vi "visionAngleDistance.vi"(11 "Limelight name":string) -> (1 "tvert":dbl, 2 "thor":dbl, 3 "ty":dbl, 4 "ta":dbl)   [LabVIEW 2019]
uses:
  TypeDefs/VisionPipeline.ctl
  ArgosLib/Signal Processing/TypeDefs/EdgeDetector_Type.ctl
  <vilib>/Rock Robotics/Network Tables/NT Write Number.vi
  <vilib>/Rock Robotics/Network Tables/NT Read Number.vi
  ArgosLib/ArgosLib.lvlib
panel:
  out "millisecond timer value":u32
  in  "pipeline control":T1=enum."NoZoom"
  in  "LED control":dbl=3.0 min=0.0 max=3.0
  out "Distance (Area-T_vertical)[In.]":dbl
  out "tx":dbl
  out "Distance (Angle.)[In.]":dbl
  in  "Target Height[in.]":dbl=100.0
  in  "Camera Height[in.]":dbl=30.0
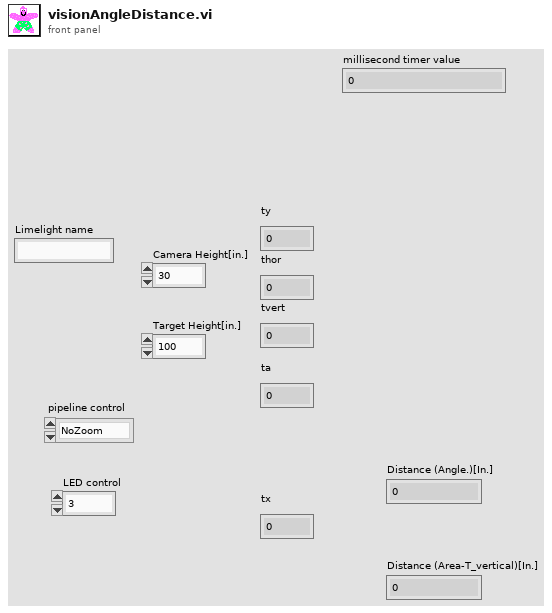
[diagram p1: front panel]
types:
  T1 = typedef "VisionPipeline.ctl" = enum16{"LEDOff", "NoZoom", "Zoom2x", "Zoom3x"}
  T2 = typedef "ArgosLib.lvlib/EdgeDetector_Type.ctl" = enum16{"RisingEdge", "FallingEdge", "Both"}
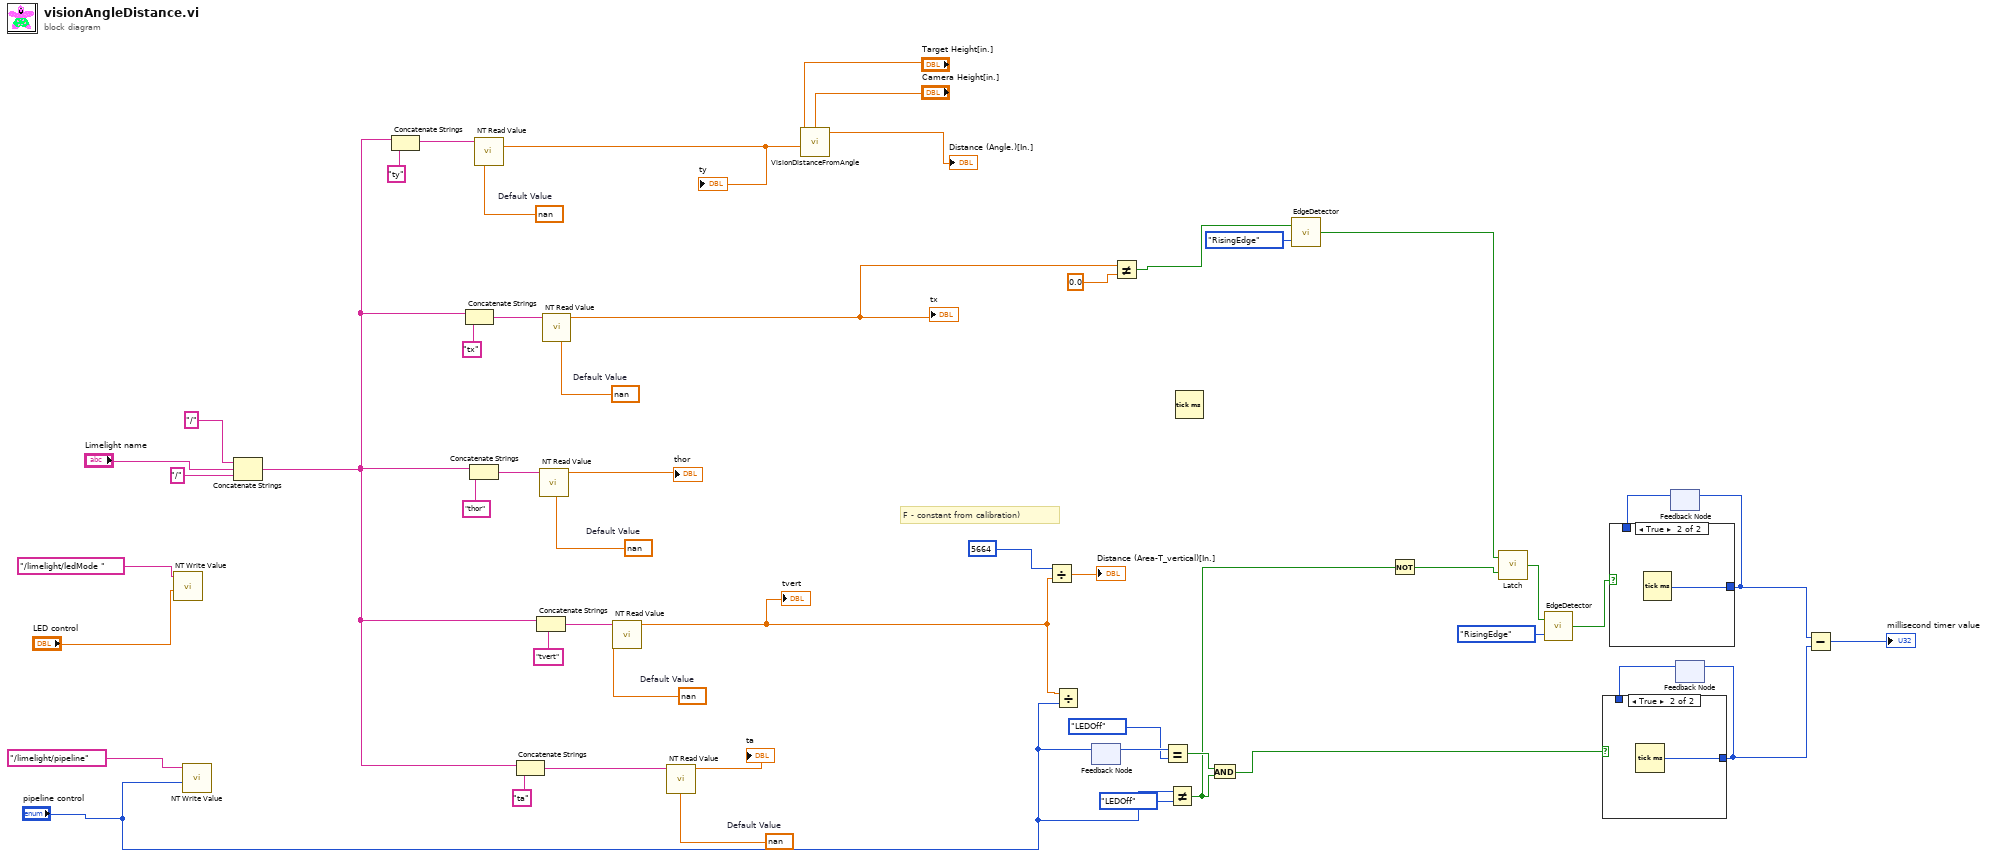
[diagram p0: block diagram]
diagram:
  w34 = nan  # Default Value
  w52 = nan  # Default Value
  w50 = nan  # Default Value
  w49 = nan  # Default Value
  w48 = nan  # Default Value
  # "F - constant from calibration)"
  n1 = call-poly <vilib>:"NT Write Value.vi"("Numeric"="LED control", "Name"="/limelight/ledMode ") -> ()  [unwired: 9 in, 1 out]
  n2 = call-poly <vilib>:"NT Write Value.vi"("Numeric"="pipeline control", "Name"="/limelight/pipeline") -> ()  [unwired: 9 in, 1 out]
  n3 = Concatenate Strings("/" ("string"), "Limelight name", "/" ("string")) -> (w30:string)
  n4 = Concatenate Strings(w30, "ty" ("Name")) -> (w32:string)
  n5 = Concatenate Strings(w30, "tx" ("Name")) -> (w36:string)
  n6 = Concatenate Strings(w30, "thor" ("Name")) -> (w43:string)
  n7 = call-poly <vilib>:"NT Read Value.vi"("Default Value"=w48, "Name"=w32) -> ("Numeric"=w29:dbl)  [unwired: 8 in, 1 out]
  "ty" <- w29
  n8 = Concatenate Strings(w30, "ta" ("Name")) -> (w39:string)
  n9 = Concatenate Strings(w30, "tvert" ("Name")) -> (w41:string)
  n10 = call-poly <vilib>:"NT Read Value.vi"("Default Value"=w49, "Name"=w43) -> ("Numeric"=→"thor":dbl)  [unwired: 8 in, 1 out]
  n11 = call-poly <vilib>:"NT Read Value.vi"("Default Value"=w34, "Name"=w36) -> ("Numeric"=w1:dbl)  [unwired: 8 in, 1 out]
  "tx" <- w1
  n12 = call-poly <vilib>:"NT Read Value.vi"("Default Value"=w50, "Name"=w41) -> ("Numeric"=w24:dbl)  [unwired: 8 in, 1 out]
  "tvert" <- w24
  n13 = call-poly <vilib>:"NT Read Value.vi"("Default Value"=w52, "Name"=w39) -> ("Numeric"=→"ta":dbl)  [unwired: 8 in, 1 out]
  n14 = call "VisionDistanceFromAngle.vi"("Ty"=w29, "Camera Height[in.]"="Camera Height[in.]", "Target Height[in.]"="Target Height[in.]") -> ("Dist. From Target[in.]"=→"Distance (Angle.)[In.]":dbl)  [unwired: 8 in]
  n15 = Divide(x=5664, y=w24) -> (x/y=→"Distance (Area-T_vertical)[In.]":dbl)
  n16 = Divide(x=w24, y="pipeline control") -> ()  [unwired: 1 out]
  n17 = feedback-in #1("pipeline control") -> ()
  n18 = feedback #1() -> (w21:T1)  [unwired: 1 in]
  n19 = Not Equal?(x=w1, y=0.0) -> (x != y?=w9:bool)
  n20 = Equal?(x=w21, y=VisionPipeline."LEDOff") -> (x = y?=w18:bool)
  n21 = Not Equal?(x="pipeline control", y=VisionPipeline."LEDOff") -> (x != y?=w3:bool)
  n22 = Tick Count (ms)() -> ()  [unwired: 1 out]
  n23 = And(x=w18, y=w3) -> (x .and. y?=w16:bool)
  n24 = call "EdgeDetector.vi"("DetectorType"=EdgeDetector_Type."RisingEdge", "Input"=w9) -> ("Edge"=w7:bool)
  n25 = Not(x=w3) -> (.not. x?=w2:bool)
  n26 = call "Latch.vi"("Reset"=w2, "Input"=w7) -> ("LatchOut"=w5:bool)
  n27 = call "EdgeDetector.vi"("DetectorType"=EdgeDetector_Type."RisingEdge", "Input"=w5) -> ("Edge"=w4:bool)
  n28 = feedback #2() -> (w13:u32)  [unwired: 1 in]
  n29 = case shown="True" w4 {
    tunnel: [w53 w54] -> w12
    tunnel: w13 -> [w53 _]
    frame False {
    }
    frame True {
      n30 = Tick Count (ms)() -> (millisecond timer value=w54:u32)
    }
  }
  n31 = feedback-in #2(w12) -> ()
  n32 = feedback #3() -> (w17:u32)  [unwired: 1 in]
  n33 = case shown="True" w16 {
    tunnel: [w55 w56] -> w11
    tunnel: w17 -> [w55 _]
    frame False {
    }
    frame True {
      n34 = Tick Count (ms)() -> (millisecond timer value=w56:u32)
    }
  }
  n35 = feedback-in #3(w11) -> ()
  n36 = Subtract(x=w12, y=w11) -> (x-y=→"millisecond timer value":u32)
